vi "Examen_IVA_01.vi"() -> ()   [LabVIEW 2020]
uses:
  <vilib>/Instr/_visa.llb/Select Event Type.ctl
  <vilib>/Instr/_visa.llb/VISA Configure Serial Port (Instr).vi
panel:
  out "Conexion":bool
  out "Sensor":string
  out "Microcontrolador":string
  out "MINIMO":i32
  out "MAXIMO":i32
  out "Voltaje":dbl
  out "Dato Leido":string
  in  "stop":bool
  out "Distancia Sensor":dynamicdata(graph)
  in  "Puerto":refnum<visa-resource-name>
  in  "parity (0:none)":enum16{"None", "Odd", "Even", "Mark", "Space"}(ring)
  in  "data bits (8)":u16=8 min=5 max=8 step=1
  in  "baud rate (9600)":u32=9600
  # "Examen 01 \nINSTRUMENTACION VIRTUAL APLICADA"
  # "Configuracion\nMicrocontrolador"
  # "Informacion"
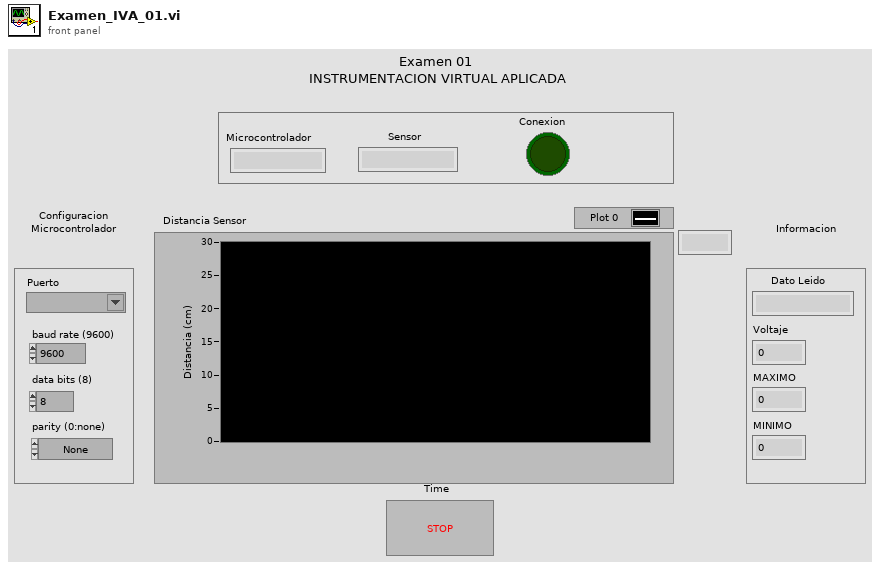
[diagram p1: front panel]
types:
  T1 = typedef "Select Event Type.ctl" = u32
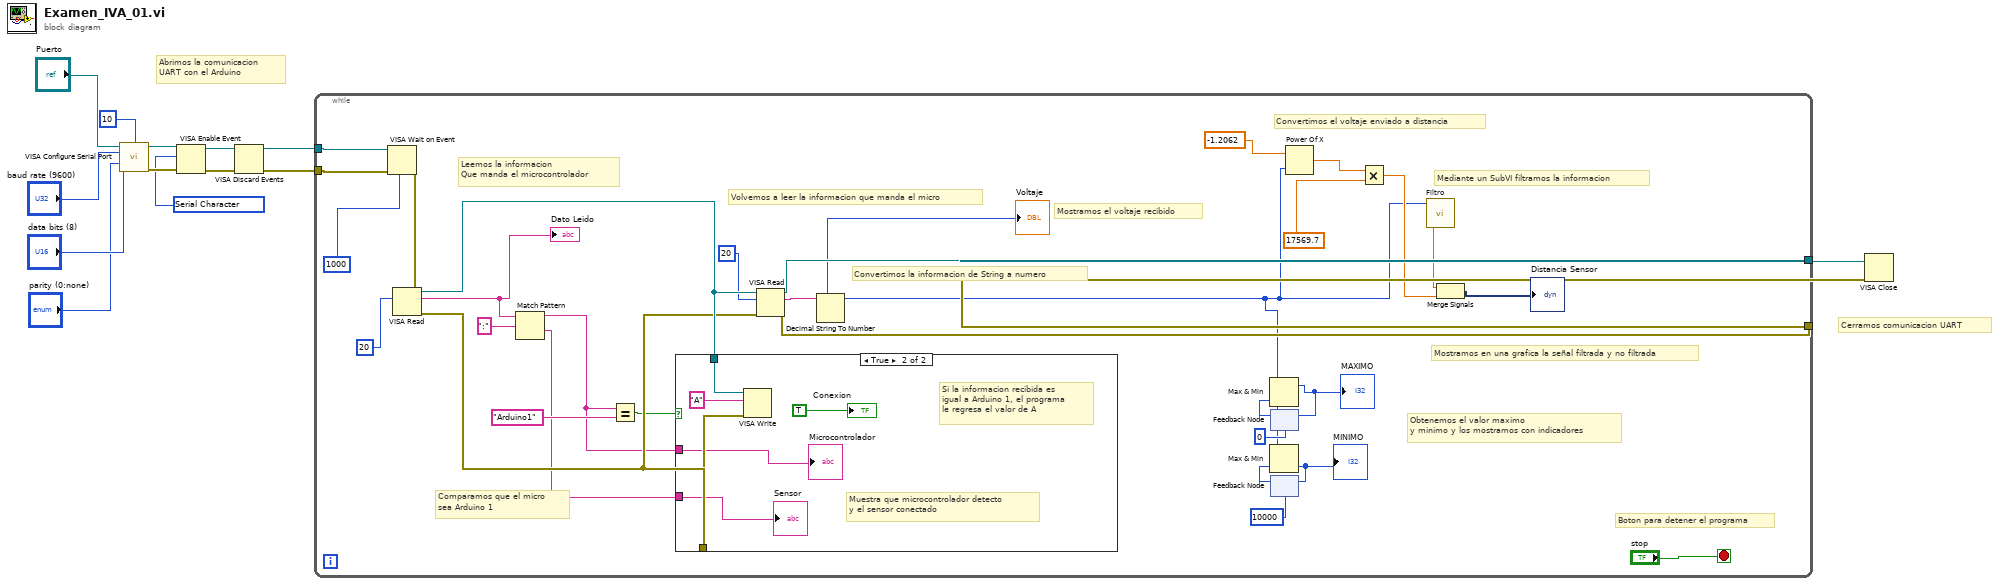
[diagram p0: block diagram]
diagram:
  w10 = T1 1073684533 items=["Service Request"=1073684491, "Trigger"=3221168138, "Clear"=1073684493, "VXI Signal"=1073684512, "VXI/VME Interrupt"=3221168161, "VXI/VME Sysfail"=1073684509, "VXI/VME Sysreset"=1073684510, "GPIB CIC"=1073684498, "GPIB Talk"=1073684499, "GPIB Listen"=1073684500, "PXI Interrupt"=1073684514, "Serial Break"=1073684515, "Serial TermChar"=1073684516, "Serial CTS"=1073684521, "Serial DSR"=1073684522, "Serial DCD"=1073684524, "Serial RI"=1073684526, "Serial Character"=1073684533, "USB Interrupt"=1073684535, "All Enabled"=1073709055] ("Event Type")
  # "Cerramos comunicacion UART"
  # "Abrimos la comunicacion\nUART con el Arduino"
  n1 = call-poly "VISA Configure Serial Port"("VISA resource name"="Puerto", "termination char\n(0xA = '\\n' = LF)"=u8 10 ("termination char\n(0xA = '\\n' = LF)"), "baud rate (9600)"="baud rate (9600)", "data bits (8)"="data bits (8)", "parity (0:none)"="parity (0:none)") -> ("VISA resource name out"=w12:refnum<visa-resource-name>, "error out"=w11:errorcluster)  [unwired: 9 in]
  n2 = VISA Enable Event(8:w11, 10:w10, 11:w12) -> (0:w8:errorcluster, 3:w9:refnum<visa-resource-name>)  [unwired: 1 in]
  n3 = VISA Discard Events(8:w8, 11:w9) -> (0:w6:errorcluster, 3:w7:refnum<visa-resource-name>)  [unwired: 2 in]
  n4 = while {
    tunnel: w7 -> [w46]
    tunnel: w6 -> [w44]
    tunnel: [w36] -> w5
    tunnel: [w35] -> w4
    stop <- "stop" stop-if-true
    # "Boton para detener el programa"
    # "Mostramos en una grafica la señal filtrada y no filtrada"
    # "Mediante un SubVI filtramos la informacion"
    # "Convertimos el voltaje enviado a distancia"
    # "Obtenemos el valor maximo \ny minimo y los mostramos con indicadores"
    # "Mostramos el voltaje recibido"
    # "Convertimos la informacion de String a numero"
    # "Volvemos a leer la informacion que manda el micro"
    # "Comparamos que el micro\nsea Arduino 1"
    # "Leemos la informacion \nQue manda el microcontrolador"
    n5 = VISA Wait on Event(7:u32 1000 ("timeout (0)"), 8:w44, 11:w46) -> (0:w42:errorcluster, 3:w39:refnum<visa-resource-name>)  [unwired: 2 in, 2 out]
    n6 = VISA Read(VISA resource name=w39, byte count=u32 20, error in (no error)=w42) -> (VISA resource name out=w38:refnum<visa-resource-name>, read buffer=w41:string, error out=w37:errorcluster)  [unwired: 1 out]
    "Dato Leido" <- w41
    n7 = Match Pattern(string=w41, regular expression=":") -> (before substring=w31:string, after substring=w25:string)  [unwired: 1 in, 2 out]
    n8 = Equal?(x=w31, y="Arduino1" ("regular expression")) -> (x = y?=w32:bool)
    n9 = case shown="True" w32 {
      tunnel: w38 -> [_ w51]
      tunnel: w37 -> [_ w50]
      tunnel: w31 -> [_ w48]
      tunnel: w25 -> [_ w47]
      frame False {
      }
      frame True {
        # "Muestra que microcontrolador detecto\ny el sensor conectado"
        # "Si la informacion recibida es \nigual a Arduino 1, el programa \nle regresa el valor de A"
        n10 = VISA Write(VISA resource name=w51, write buffer="A", error in (no error)=w50) -> ()  [unwired: 3 out]
        "Conexion" <- TRUE
        "Microcontrolador" <- w48
        "Sensor" <- w47
      }
    }
    n11 = VISA Read(VISA resource name=w38, byte count=u32 20, error in (no error)=w37) -> (VISA resource name out=w35:refnum<visa-resource-name>, read buffer=w30:string, error out=w36:errorcluster)  [unwired: 1 out]
    n12 = Decimal String To Number(string=w30) -> (number=w15:i32)  [unwired: 2 in, 1 out]
    "Voltaje" <- w15
    n13 = feedback #1(0) -> (w29:i32)
    n14 = Max & Min(x=w15, y=w29) -> (max(x,y)=w24:i32)  [unwired: 1 out]
    "MAXIMO" <- w24
    n15 = feedback-in #1(w24) -> ()
    n16 = feedback #2(10000) -> (w28:i32)
    n17 = Max & Min(x=w15, y=w28) -> (min(x,y)=w23:i32)  [unwired: 1 out]
    "MINIMO" <- w23
    n18 = feedback-in #2(w23) -> ()
    n19 = Power Of X(1:w15, 2:-1.2062 ("x")) -> (0:w18:dbl)
    n20 = Multiply(x=w18, y=17569.7) -> (x*y=w16:dbl)
    n21 = call "Filtro.vi"("Numeric in"=w15) -> ("Numeric out"=w21:dbl)  [unwired: 10 in]
    n22 = Merge Signals(w21, w16) -> (→"Distancia Sensor":dynamicdata)
  }
  n23 = VISA Close(VISA resource name=w4, error in (no error)=w5) -> ()  [unwired: 1 out]
